vi "高亮当前行.vi"(10 "Row":i32, 11 "Table输入":refnum<vi>) -> (3 "引用输出":refnum<vi>)   [LabVIEW 2014]
uses:
  <vilib>/Utility/miscctls.llb/LVRowAndColumnTypeDef.ctl
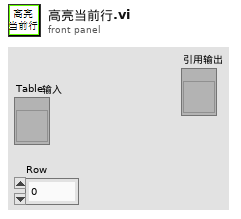
[diagram p1: front panel]
types:
  T1 = typedef "LVRowAndColumnTypeDef.ctl" = cluster{"Row":i32, "Column":i32}
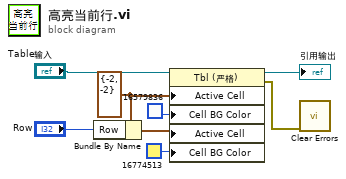
[diagram p0: block diagram]
diagram:
  w4 = T1 {"Row"=-2, "Column"=-2} ("Active Cell:Active Cell")
  n1 = Bundle By Name(cluster=w4, "Row"="Row") -> (w5:T1)
  n2 = property on="属性节点" class="Tbl (严格)"(reference="Table输入", "Active Cell"=w4, "Cell BG Color"=u32 16579836, "Active Cell"=w5, "Cell BG Color"=u32 16774513) -> (reference out=→"引用输出":refnum<vi>, error out=w1:errorcluster)  [unwired: 1 in]
  n3 = call <vilib>:"Clear Errors.vi"("error in (no error)"=w1) -> ()  [unwired: 5 in, 2 out]
